vi "Implementation Path.vi"() -> (3 "All Files in Dir":path[](array[path]))   [LabVIEW 2020, in "FGen.lvlib"]
uses:
  FGen.lvlib
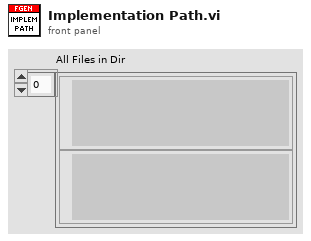
[diagram p1: front panel]
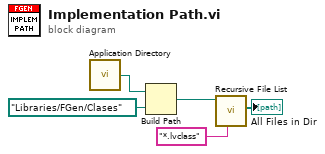
[diagram p0: block diagram]
diagram:
  n1 = call <vilib>:"Application Directory.vi"() -> ("Application Directory"=w1:path)
  n2 = Build Path(base path=w1, name or relative path=path "Libraries/FGen/Clases") -> (appended path=w3:path)
  n3 = call <vilib>:"Recursive File List.vi"("pattern"="*.lvclass", "Folder Path"=w3) -> ("All Files in Dir"=→"All Files in Dir":path[])  [unwired: 5 in, 4 out]
